vi "基础价格.vi"(8 "error in (no error)":errorcluster caption="错误输入（无错误）", 11 "醇香奶茶 输入":refnum<class "醇香奶茶.lvclass">) -> (0 "error out":errorcluster caption="错误输出", 2 "基础价格":dbl, 3 "醇香奶茶 输出":refnum<class "醇香奶茶.lvclass">)   [LabVIEW 2016, in "醇香奶茶.lvclass"]
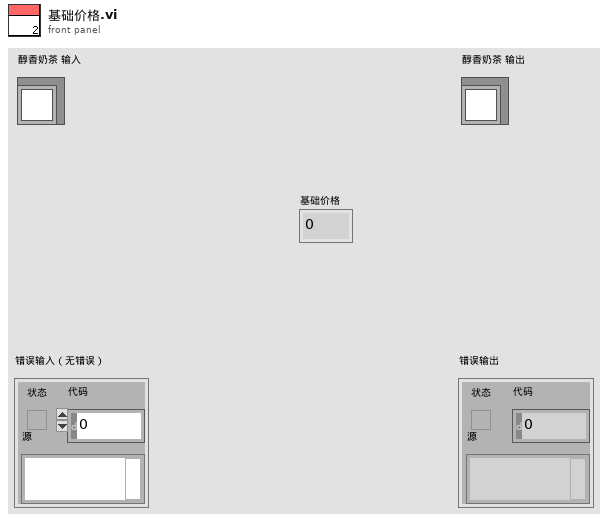
[diagram p1: front panel]
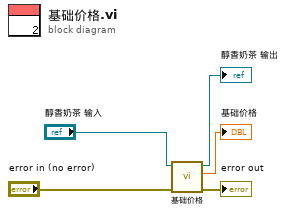
[diagram p0: block diagram]
diagram:
  n1 = call-parent "基础价格.vi"("error in (no error)"="error in (no error)", "奶茶 输入"="醇香奶茶 输入") -> ("error out"=→"error out":errorcluster, "基础价格"=→"基础价格":dbl, "奶茶 输出"=→"醇香奶茶 输出":refnum<class "醇香奶茶.lvclass">)  [unwired: 7 in]
